vi "Register Broadcast(2x parallel).vi"() -> ()   [LabVIEW 2020, in "TCPRouter ClientAPI Examples.lvlib"]
uses:
  _addons/TCP-Router/ClientAPI/Def-TCP-Router Status Data.ctl
  97d7a57c-b8d6-491e-bd00-19fa11dae530.vi
  7e38bf89-2462-47fa-b6f6-5b46729ec3b2.vi
  769d4601-277e-42af-bd46-57be9b140e3e.vi
  b3b63605-1016-4be4-a788-12e3256b011c.vi
  <userlib>/_NEVSTOP/Communicable State Machine(CSM)/addons/API-String-Arugments-Support/_Support/Convert API String Arguments to Data(variant).vi
  TCPRouter ClientAPI Examples.lvlib
  _addons/TCP-Router/ClientAPI/TcpRouter-Client.lvclass
panel:
  out "Waveform Chart 2":dbl(graph)
  out "Waveform Chart":dbl(graph)
  out "error out 2":errorcluster
  out "error out":errorcluster
  out "element 2":T1
  out "current time 2":timestamp
  out "# elements in queue 2":i32
  out "# elements in queue":i32
  out "current time":timestamp
  out "element":T1
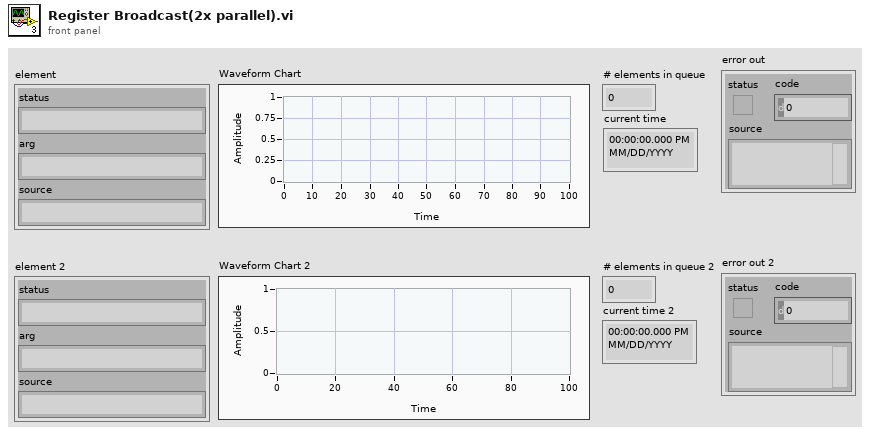
[diagram p1: front panel]
types:
  T1 = typedef "CSM-TCP-Router.lvlib/TcpRouter-Client.lvclass/Def-TCP-Router Status Data.ctl" = cluster{"status":string, "arg":string, "source":string}
  T2 = cluster{"IP Address":string, "Port":u16, "ConnectTMO":i32}
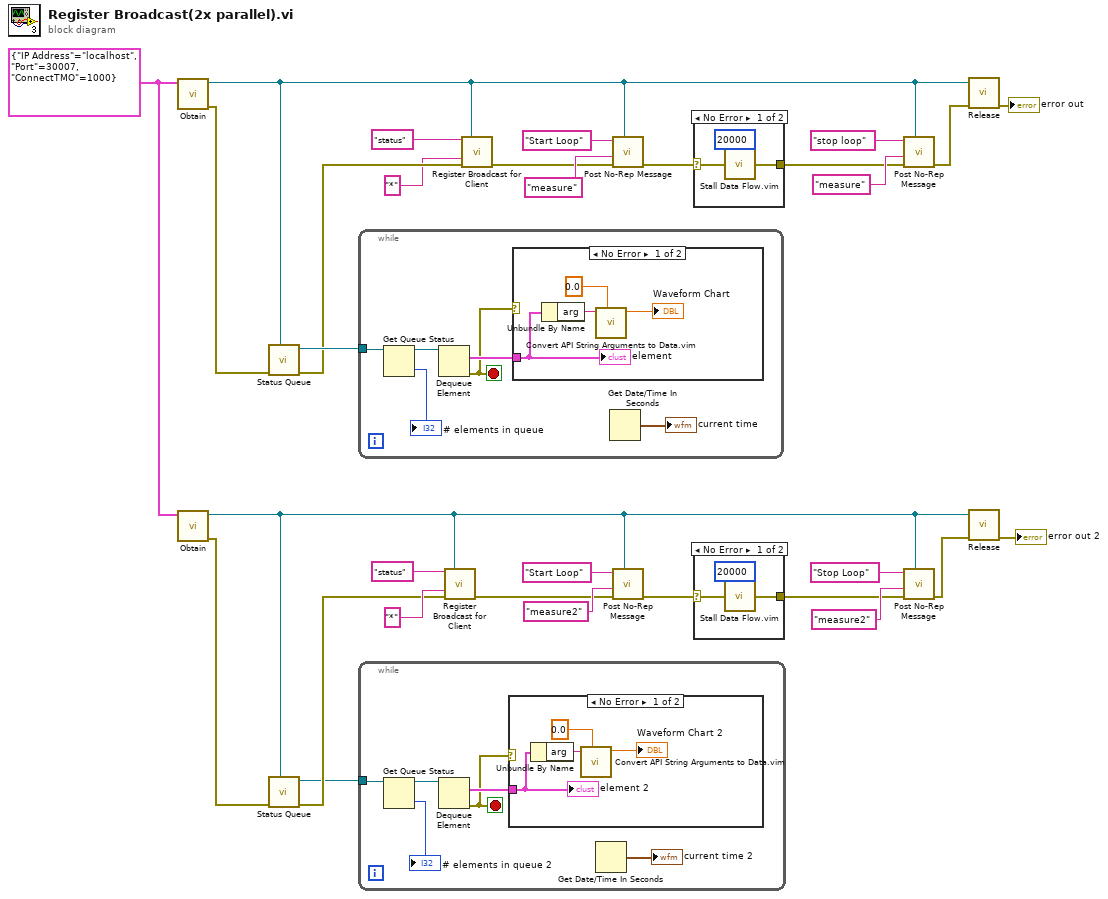
[diagram p0: block diagram]
diagram:
  w8 = T2 {"IP Address"="localhost", "Port"=30007, "ConnectTMO"=1000} ("Connection")
  n1 = call "Obtain.vi"("Connection"=w8) -> ("error out"=w25:errorcluster, "TcpRouter-Client out"=w7:refnum<class "TcpRouter-Client.lvclass">)  [unwired: 9 in]
  n2 = call "Obtain.vi"("Connection"=w8) -> ("error out"=w12:errorcluster, "TcpRouter-Client out"=w22:refnum<class "TcpRouter-Client.lvclass">)  [unwired: 9 in]
  n3 = call "Status Queue.vi"("TcpRouter-Client in"=w7, "error in (no error)"=w25) -> ("error out"=w5:errorcluster, "StatusQueue"=w26:refnum<queue>)  [unwired: 8 in]
  n4 = call "Status Queue.vi"("TcpRouter-Client in"=w22, "error in (no error)"=w12) -> ("error out"=w13:errorcluster, "StatusQueue"=w10:refnum<queue>)  [unwired: 8 in]
  n5 = while {
    tunnel: w26 -> [w37]
    stop <- w32 stop-if-true
    n6 = Get Queue Status(queue=w37) -> (queue out=w35:refnum<queue>, # elements in queue=→"# elements in queue":i32)  [unwired: 2 in, 6 out]
    n7 = Dequeue Element(queue=w35) -> (element=w33:T1, error out=w32:errorcluster)  [unwired: 2 in, 2 out]
    n8 = case shown="No Error" w32 {
      tunnel: w33 -> [w38 _]
      frame No Error {
        n9 = Unbundle By Name(w38) -> ("arg"=w41:string)
        n10 = call "Convert API String Arguments to Data.vim"("Reference Type"=0.0, "API String"=w41) -> ("Data"=→"Waveform Chart":dbl)  [unwired: 6 in, 1 out]
        "element" <- w38
      }
      frame Error {
      }
    }
    n11 = Get Date/Time In Seconds() -> (seconds since 1Jan1904=→"current time":timestamp)
  }
  n12 = while {
    tunnel: w10 -> [w47]
    stop <- w42 stop-if-true
    n13 = Get Queue Status(queue=w47) -> (queue out=w45:refnum<queue>, # elements in queue=→"# elements in queue 2":i32)  [unwired: 2 in, 6 out]
    n14 = Dequeue Element(queue=w45) -> (element=w43:T1, error out=w42:errorcluster)  [unwired: 2 in, 2 out]
    n15 = case shown="No Error" w42 {
      tunnel: w43 -> [w51 _]
      frame No Error {
        n16 = Unbundle By Name(w51) -> ("arg"=w50:string)
        n17 = call "Convert API String Arguments to Data.vim"("Reference Type"=0.0, "API String"=w50) -> ("Data"=→"Waveform Chart 2":dbl)  [unwired: 6 in, 1 out]
        "element 2" <- w51
      }
      frame Error {
      }
    }
    n18 = Get Date/Time In Seconds() -> (seconds since 1Jan1904=→"current time 2":timestamp)
  }
  n19 = call "Register Broadcast for Client.vi"("Status"="status" ("CSM Name"), "TcpRouter-Client in"=w22, "CSM Name"="*" ("Source CSM Name (* as Default)"), "error in (no error)"=w13) -> ("error out"=w11:errorcluster)  [unwired: 10 in, 1 out]
  n20 = call "Register Broadcast for Client.vi"("Status"="status" ("CSM Name"), "TcpRouter-Client in"=w7, "CSM Name"="*" ("Source CSM Name (* as Default)"), "error in (no error)"=w5) -> ("error out"=w6:errorcluster)  [unwired: 10 in, 1 out]
  n21 = call "Post No-Rep Message.vi"("TcpRouter-Client in"=w7, "error in (no error)"=w6, "Target Module"="measure", "State"="Start Loop") -> ("error out"=w24:errorcluster)  [unwired: 7 in]
  n22 = call "Post No-Rep Message.vi"("TcpRouter-Client in"=w22, "error in (no error)"=w11, "Target Module"="measure2", "State"="Start Loop") -> ("error out"=w18:errorcluster)  [unwired: 7 in]
  n23 = case shown="No Error" w24 {
    selector: w24 -> [w52 w55]
    tunnel: [w54 w55] -> w27
    frame No Error {
      n24 = call "Stall Data Flow.vim"("value in"=w52, "milliseconds to wait"=u32 20000) -> ("value out"=w54:errorcluster)  [unwired: 1 out]
    }
    frame Error {
    }
  }
  n25 = case shown="No Error" w18 {
    selector: w18 -> [w56 w59]
    tunnel: [w58 w59] -> w9
    frame No Error {
      n26 = call "Stall Data Flow.vim"("value in"=w56, "milliseconds to wait"=u32 20000) -> ("value out"=w58:errorcluster)  [unwired: 1 out]
    }
    frame Error {
    }
  }
  n27 = call "Post No-Rep Message.vi"("TcpRouter-Client in"=w7, "error in (no error)"=w27, "Target Module"="measure", "State"="stop loop") -> ("error out"=w23:errorcluster)  [unwired: 7 in]
  n28 = call "Post No-Rep Message.vi"("TcpRouter-Client in"=w22, "error in (no error)"=w9, "Target Module"="measure2", "State"="Stop Loop") -> ("error out"=w21:errorcluster)  [unwired: 7 in]
  n29 = call "Release.vi"("error in (no error)"=w23, "TcpRouter-Client in"=w7) -> ("error out"=→"error out":errorcluster)  [unwired: 9 in]
  n30 = call "Release.vi"("error in (no error)"=w21, "TcpRouter-Client in"=w22) -> ("error out"=→"error out 2":errorcluster)  [unwired: 9 in]
